vi "autohideVScrollbar.vi"(8 "error in (no error)":errorcluster, 10 "Table in":refnum<vi>, 11 "State":T1={"logTable"=refnum, "max items"=500, "displaydata"=[], "data"=[], "Auto Scroll"=TRUE, "current item"=500, "col headers"=[], "Add to Top"=TRUE, "Auto resize"=TRUE, "col size"=[], "filters"=[], "color cells"=[]}) -> (0 "error out":errorcluster, 2 "Table out":refnum<vi>, 3 "State (dup)":T1={"logTable"=refnum, "max items"=500, "displaydata"=[], "data"=[], "Auto Scroll"=TRUE, "current item"=500, "col headers"=[], "Add to Top"=TRUE, "Auto resize"=TRUE, "col size"=[], "filters"=[], "color cells"=[]})   [LabVIEW 2013, in "UI-DisplayTable(dev).xctl"]
uses:
  UI-DisplayTable(dev).xctl
  State.ctl
  DEF-Filter.ctl
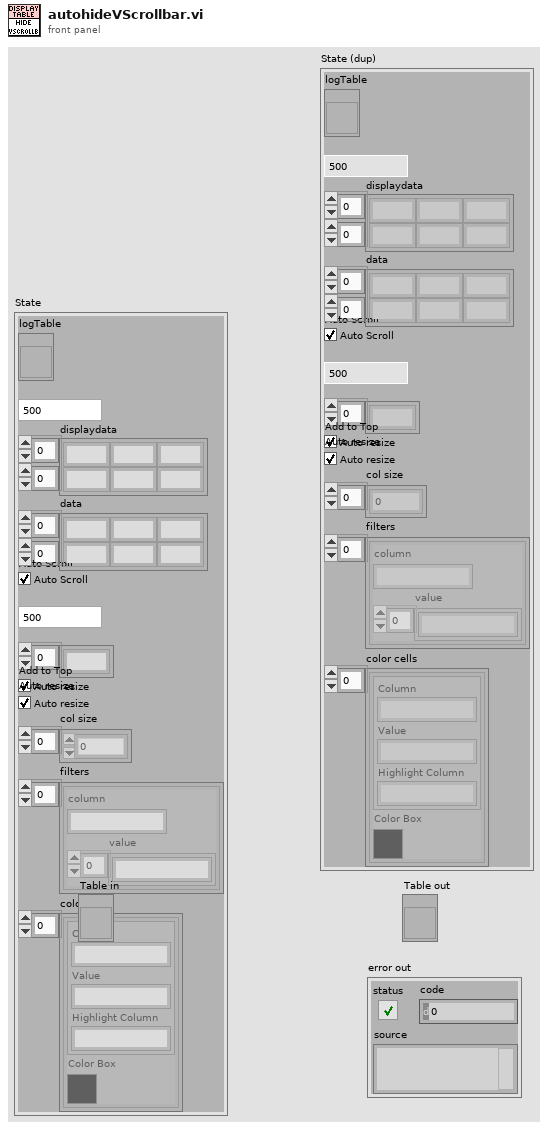
[diagram p1: front panel]
types:
  T1 = typedef "UI-DisplayTable(dev).xctl/State.ctl" = cluster{"logTable":refnum<vi>, "max items":i32, "displaydata":string[][], "data":string[][], "Auto Scroll":bool, "current item":i32, "col headers":string[], "Add to Top":bool, "Auto resize":bool, "col size":i32[], "filters":T2[], "color cells":cluster{"color cell":cluster{"Column":string, "Value":string, "Highlight Column":string}, "Color Box":u32}[]}
  T2 = typedef "UI-DisplayTable(dev).xctl/DEF-Filter.ctl" = cluster{"column":string, "value":string[]}
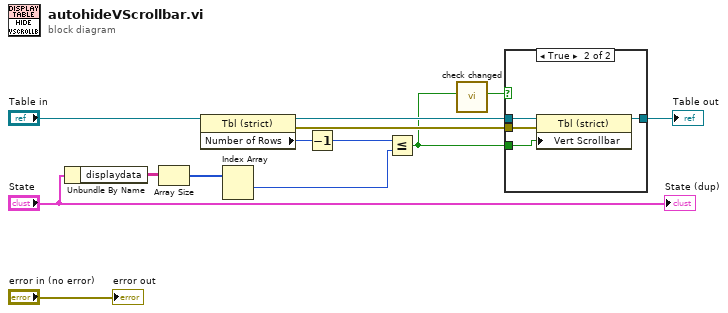
[diagram p0: block diagram]
diagram:
  n1 = Unbundle By Name("State") -> ("displaydata"=w6:string[][])
  n2 = Array Size(array=w6) -> (size(s)=w5:i32[])
  n3 = property class="Tbl (strict)"(reference="Table in") -> (reference out=w9:refnum<vi>, error out=w8:errorcluster, "Number of Rows"=w7:u32)  [unwired: 1 in]
  n4 = Index Array(array=w5) -> (element #1=w4:i32)  [unwired: 2 in, 1 out]
  n5 = Decrement(x=w7) -> (x-1=w3:u32)
  n6 = Less Or Equal?(x=w3, y=w4) -> (x <= y?=w2:bool)
  n7 = call "check changed.vi"("data"=w2) -> ("changed?"=w1:bool)  [unwired: 9 in, 1 out]
  n8 = case shown="True" w1 {
    tunnel: [w14 w18] -> w11
    tunnel: w9 -> [w14 w17]
    tunnel: w8 -> [_ w16]
    tunnel: w2 -> [_ w15]
    frame False {
    }
    frame True {
      n9 = property class="Tbl (strict)"(reference=w17, error in=w16, "Vert Scrollbar"=w15) -> (reference out=w18:refnum<vi>)  [unwired: 1 out]
    }
  }
  "Table out" <- w11
  "error out" <- "error in (no error)"
  "State (dup)" <- "State"
